vi "Load App.vi"(8 "error in (no error)":errorcluster, 11 "Controller Actor.lvlib:Controller.lvclass":refnum<class "Controller.lvclass">) -> (0 "error out":errorcluster)   [LabVIEW 2016, in "Controller Actor.lvlib" / "Controller.lvclass"]
uses:
  <userlib>/Common Components/Controller/Controller.lvclass
  C:/Program Files (x86)/National Instruments/LabVIEW 2016/vi.lib/ActorFramework/Actor/Actor.lvclass
  <vilib>/ActorFramework/Message Queue/Message Queue.lvclass/Message Queue.ctl
  <vilib>/ActorFramework/Actor/Actor.lvclass
  <vilib>/ActorFramework/Message Queue/Message Queue.lvclass
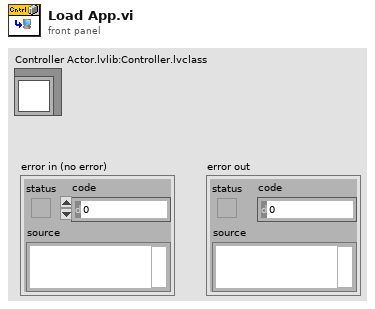
[diagram p1: front panel]
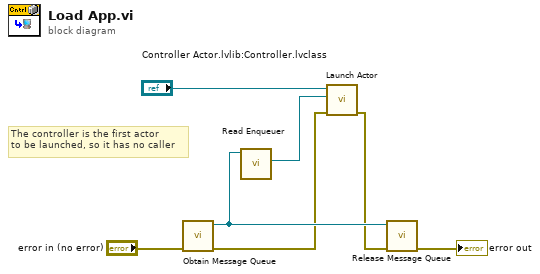
[diagram p0: block diagram]
diagram:
  # "The controller is the first actor\nto be launched, so it has no caller"
  n1 = call <vilib>:"Obtain Message Queue.vi"("error in (no error)"="error in (no error)") -> ("error out"=w6:errorcluster, "Message Queue"=w7:refnum<class "Message Queue.lvclass">)  [unwired: 9 in]
  n2 = call <vilib>:"Read Enqueuer.vi"("Message Queue"=w7) -> ("Message Enqueuer"=w4:refnum<class "Message Enqueuer.lvclass">)  [unwired: 10 in]
  n3 = call <vilib>:"Launch Actor.vi"("error in (no error)"=w6, "Actor-to-Caller Enqueuer"=w4, "Actor"="Controller Actor.lvlib:Controller.lvclass") -> ("error out"=w5:errorcluster)  [unwired: 7 in, 1 out]
  n4 = call <vilib>:"Release Message Queue.vi"("error in (no error)"=w5, "Message Queue"=w7) -> ("error out"=→"error out":errorcluster)  [unwired: 8 in, 1 out]
